vi "Red's Auto Clicker.vi"(8 "error in (no error)":errorcluster) -> (0 "error out":errorcluster)   [LabVIEW 2020]
doc: "Presents an interface to create, edit, save, and execute user-defined macros."
uses:
  CTLs/State Data.ctl
  CTLs/Macro Cluster V3.ctl
  CTLs/Macro Config V3.ctl
  CTLs/Step V3.ctl
  CTLs/Step Type V3.ctl
  CTLs/Hotkey Values.ctl
  CTLs/Refs.ctl
  <vilib>/Utility/miscctls.llb/LVRowAndColumnUnsignedTypeDef.ctl
  CTLs/FGV Actions.ctl
  CTLs/Hotkey Type.ctl
  fa5aba67-e91f-4216-ac5c-c17457851557.vi
  bd503c13-d10c-440e-ab5e-4e60baef5deb.vi
  <vilib>/Utility/inputDevices.llb/closeKeyboard.vi
  SubVIs/FaKI State Machine/FaKI State Machine.lvlib
panel:
  out "Status":string
  in  "Add Step 2":bool
  in  "Dbl Click":T1
  in  "Macro Steps":i32(listbox)
  out "Abort Hotkey":string caption="Abort Hotkey:"
  out "Metadata":string
  in  "Description":string
  out "Resolutions":cluster{"Width":i16, "Height":i16}[](array[cluster])
  out "n Monitors":i32
  in  "Settings":bool
  in  "Export":bool
  in  "Import":bool
  out "Macro Hotkey":string caption="Macro Hotkey:"
  in  "Delete":bool
  in  "Start/Stop":bool
  in  "N":i32 caption="Times to Repeat\n(-1 = indefinitely)" min=-1
  in  "Activation Type":enum32{"Hotkey", "Automatic"}(radio)
  out "Row":i32
  in  "Clear Steps":bool
  in  "Delete Step":bool
  in  "Insert Step":bool
  in  "Add Step":bool
  in  "Modify Step":bool
  in  "Exit":bool
  in  "Save":bool
  in  "Restore":bool
  in  "Help":bool
  in  "Macro Name":string(combo)
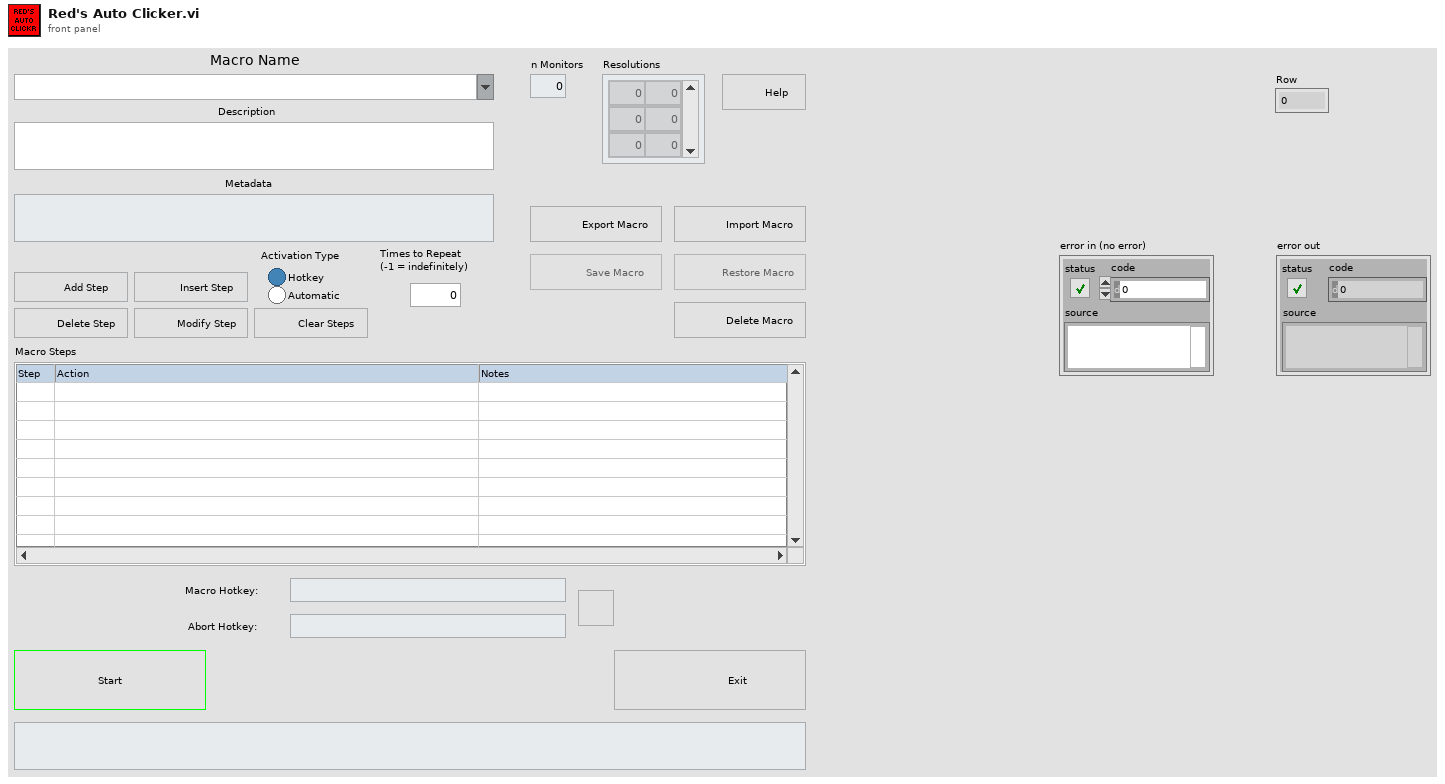
[diagram p1: front panel]
types:
  T1 = cluster{"Insert Before":bool, "Insert After":bool, "Modify Step 2":bool, "Delete Step 2":bool}
  T2 = typedef "LVPoint32TypeDef.ctl" = cluster{"Horizontal":i32, "Vertical":i32}
  T3 = enum32{"Invalid", "Standard", "Closed", "Hidden", "Minimized", "Maximized"}
  T4 = enum32{"invalid app kind", "Development System", "Run Time System", "Student Edition", "Embedded LabVIEW", "Evaluation", "Custom"}
  T5 = typedef "State Data.ctl" = cluster{"Core":cluster{"Current VI Reference":refnum<vi>, "Close Panel on Exit?":bool}, "Macro":cluster{"New":T6, "Saved":T6, "Name":string}, "Step":i32, "n":i32, "Hotkey Values":T10, "Keyboard":refnum<k1>, "Macro Active?":bool, "Macro Names":string[], "Rcount":i32, "Refs":T11, "Resolutions":cluster{"Width":i16, "Height":i16}[], "App Data Dir":path, "Start Time":timestamp}
  T6 = typedef "Macro Cluster V3.ctl" = cluster{"Config":T7, "Steps":T8[]}
  T7 = typedef "Macro Config V3.ctl" = cluster{"Schema Version":string, "Activation Type":enum32{"Hotkey", "Automatic"}, "N":i32, "Description":string, "Resolutions":cluster{"Width":i16, "Height":i16}[], "Date Created":timestamp, "Date Updated":timestamp}
  T8 = typedef "Step V3.ctl" = cluster{"Type":T9, "X":i32, "Y":i32, "Delay":i32, "Key":u8, "Repeat":i32, "RClick?":bool, "App/Window Name":string, "Notes":string}
  T9 = typedef "Step Type V3.ctl" = enum16{"Mouse Move", "Mouse Click", "Key Press", "Wait", "Mouse Down", "Mouse Up", "Key Down", "Key Up", "Run Application", "Maximize Window", "Restore Window", "Minimize Window", "Close Window", "Bring Window to Front", "Send Window to Back"}
  T10 = typedef "Hotkey Values.ctl" = cluster{"Macro Hotkey":enum16{"0", "1", "2", "3", "4", "5", "6", "7", "8", "9", "A", "B", "C", "D", "E", "F", "G", "H", "I", "J", "K", "L", "M", "N", "O", "P", "Q", "R", "S", "T", "U", "V", "W", "X", "Y", "Z", "F1", "F2", "F3", "F4", "F5", "F6", "F7", "F8", "F9", "F10", "F11", "F12", "F13", "F14", "F15", "ADD", "BACK", "BACKSLASH", "CAPITAL", "COMMA", "DECIMAL", "DELETE", "DIVIDE", "DOWN", "END", "EQUALS", "ESCAPE", "GRAVE (`)", "HOME", "INSERT", "LBRACKET", "LCONTROL", "LEFT", "L ALT", "LSHIFT", "LWIN", "MINUS", "MULTIPLY", "NEXT", "NUMLOCK", "NUMPAD_0", "NUMPAD_1", "NUMPAD_2", "NUMPAD_3", "NUMPAD_4", "NUMPAD_5", "NUMPAD_6", "NUMPAD_7", "NUMPAD_8", "NUMPAD_9", "PAUSE", "PERIOD", "PRIOR (PG UP)", "RBRACKET", "RCONTROL", "RETURN", "RIGHT", "R ALT", "RSHIFT", "RWIN", "SCROLL", "SEMICOLON", "SLASH", "SPACE", "SUBTRACT", "TAB", "UP", "ENTER (num pad)", "' (quote)"}[], "Abort Hotkey":enum16{"0", "1", "2", "3", "4", "5", "6", "7", "8", "9", "A", "B", "C", "D", "E", "F", "G", "H", "I", "J", "K", "L", "M", "N", "O", "P", "Q", "R", "S", "T", "U", "V", "W", "X", "Y", "Z", "F1", "F2", "F3", "F4", "F5", "F6", "F7", "F8", "F9", "F10", "F11", "F12", "F13", "F14", "F15", "ADD", "BACK", "BACKSLASH", "CAPITAL", "COMMA", "DECIMAL", "DELETE", "DIVIDE", "DOWN", "END", "EQUALS", "ESCAPE", "GRAVE (`)", "HOME", "INSERT", "LBRACKET", "LCONTROL", "LEFT", "L ALT", "LSHIFT", "LWIN", "MINUS", "MULTIPLY", "NEXT", "NUMLOCK", "NUMPAD_0", "NUMPAD_1", "NUMPAD_2", "NUMPAD_3", "NUMPAD_4", "NUMPAD_5", "NUMPAD_6", "NUMPAD_7", "NUMPAD_8", "NUMPAD_9", "PAUSE", "PERIOD", "PRIOR (PG UP)", "RBRACKET", "RCONTROL", "RETURN", "RIGHT", "R ALT", "RSHIFT", "RWIN", "SCROLL", "SEMICOLON", "SLASH", "SPACE", "SUBTRACT", "TAB", "UP", "ENTER (num pad)", "' (quote)"}[]}
  T11 = typedef "Refs.ctl" = cluster{"Name":refnum<vi>, "Description":refnum<vi>, "Import":refnum<vi>, "Export":refnum<vi>, "Delete":refnum<vi>, "Restore":refnum<vi>, "Save":refnum<vi>, "Start":refnum<vi>, "Steps":refnum<vi>, "Simple Refs":refnum<vi>[]}
  T12 = enum8{"Enabled", "Disabled", "Disabled and Grayed Out"}
  T13 = typedef "LVRowAndColumnUnsignedTypeDef.ctl" = cluster{"Row":u32, "Column":u32}
  T14 = typedef "Hotkey Type.ctl" = enum16{"Macro Hotkey", "Abort Hotkey"}
  T15 = typedef "FGV Actions.ctl" = enum16{"Read", "Write"}
  T16 = cluster{"Current VI Reference":refnum<vi>, "Close Panel on Exit?":bool}
  T17 = enum16{"0", "1", "2", "3", "4", "5", "6", "7", "8", "9", "A", "B", "C", "D", "E", "F", "G", "H", "I", "J", "K", "L", "M", "N", "O", "P", "Q", "R", "S", "T", "U", "V", "W", "X", "Y", "Z", "F1", "F2", "F3", "F4", "F5", "F6", "F7", "F8", "F9", "F10", "F11", "F12", "F13", "F14", "F15", "ADD", "BACK", "BACKSLASH", "CAPITAL", "COMMA", "DECIMAL", "DELETE", "DIVIDE", "DOWN", "END", "EQUALS", "ESCAPE", "GRAVE (`)", "HOME", "INSERT", "LBRACKET", "LCONTROL", "LEFT", "L ALT", "LSHIFT", "LWIN", "MINUS", "MULTIPLY", "NEXT", "NUMLOCK", "NUMPAD_0", "NUMPAD_1", "NUMPAD_2", "NUMPAD_3", "NUMPAD_4", "NUMPAD_5", "NUMPAD_6", "NUMPAD_7", "NUMPAD_8", "NUMPAD_9", "PAUSE", "PERIOD", "PRIOR (PG UP)", "RBRACKET", "RCONTROL", "RETURN", "RIGHT", "R ALT", "RSHIFT", "RWIN", "SCROLL", "SEMICOLON", "SLASH", "SPACE", "SUBTRACT", "TAB", "UP", "ENTER (num pad)", "' (quote)"}[]
  T18 = typedef "LVAllMonitorsDisplayTypeDef.ctl" = cluster{"Bounds":cluster{"Left":i16, "Top":i16, "Right":i16, "Bottom":i16}, "Depth":i16}[]
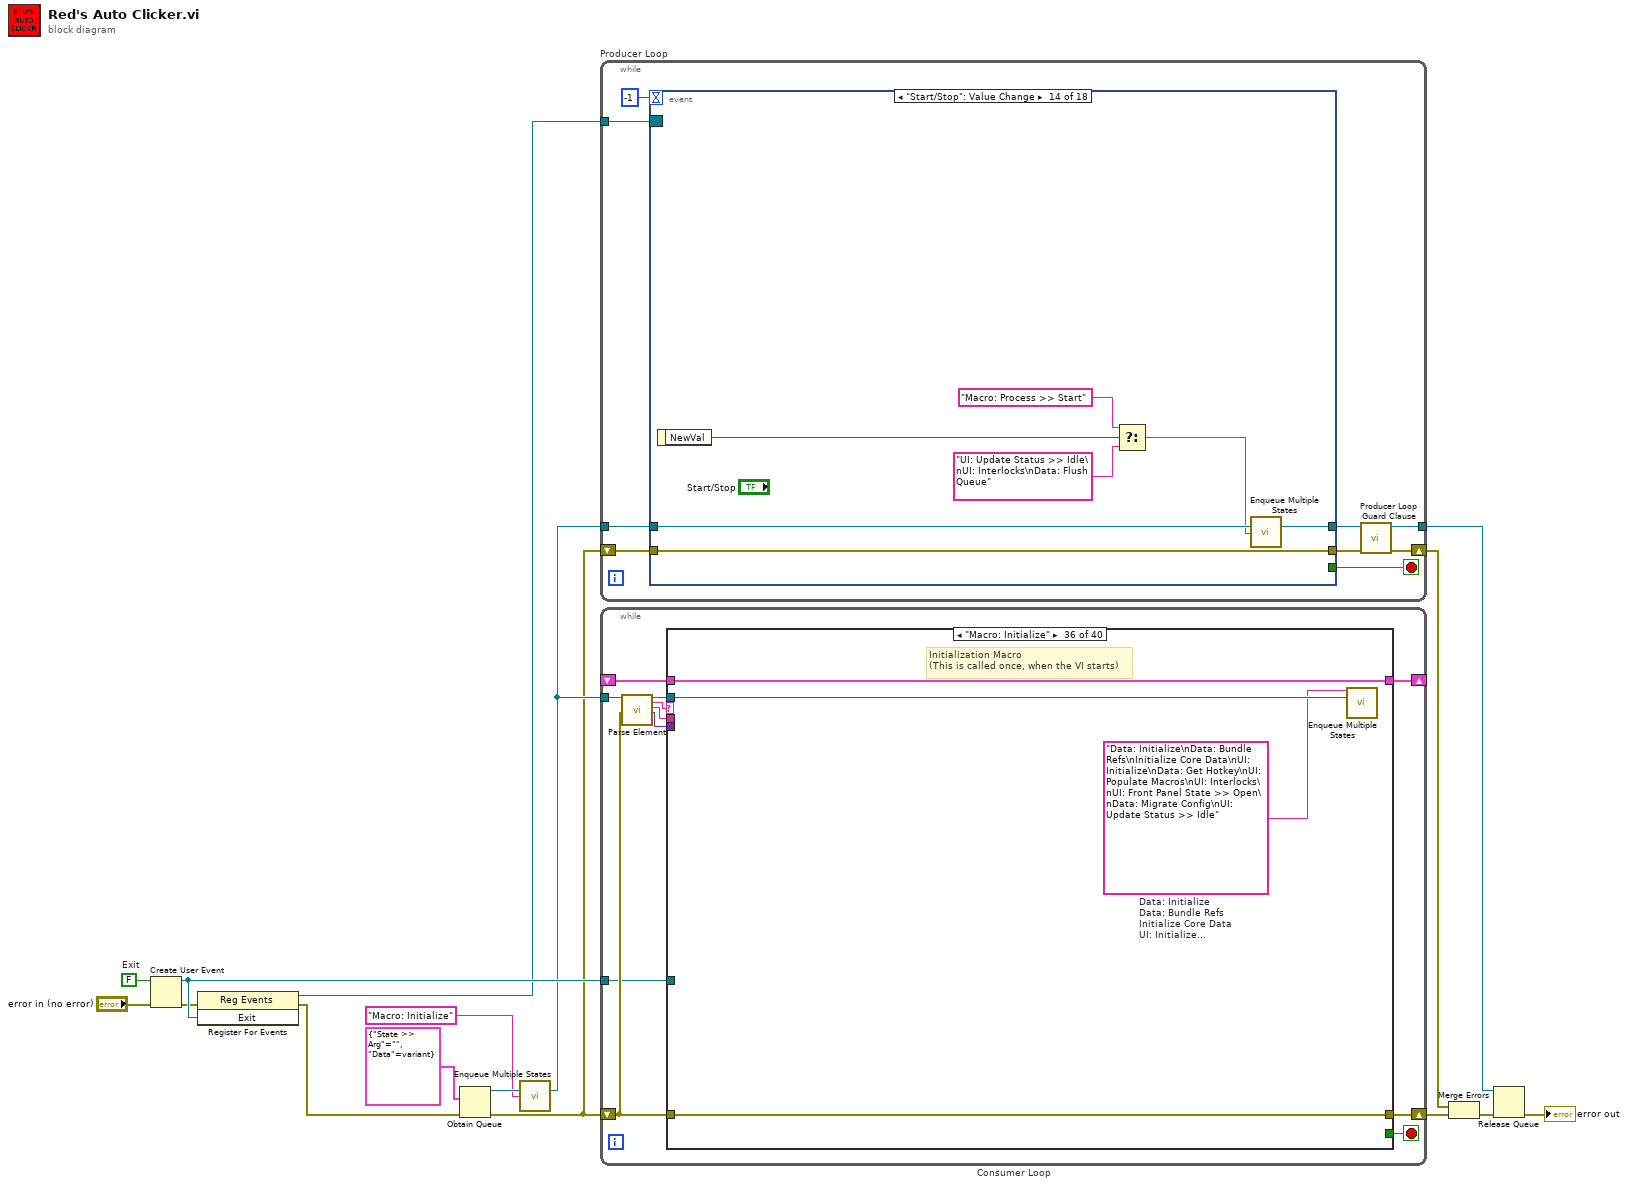
[diagram p0: block diagram]
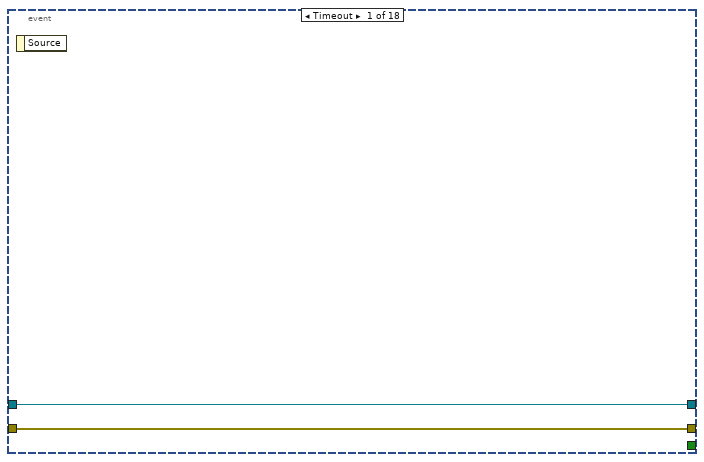
[diagram p2: hidden frame]
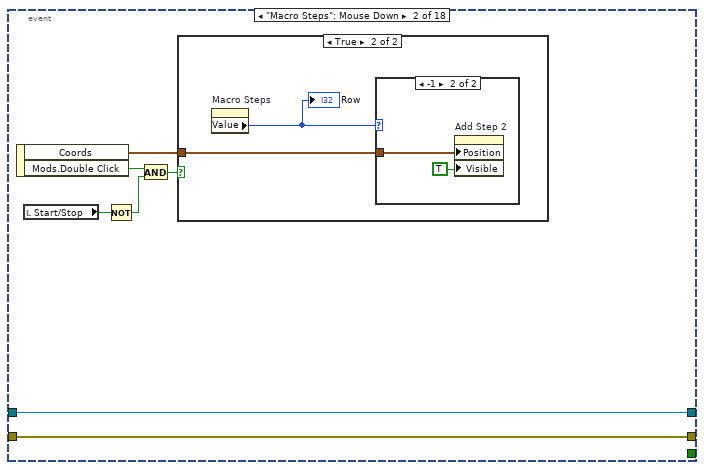
[diagram p3: hidden frame]
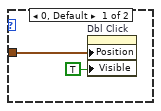
[diagram p5: hidden frame]
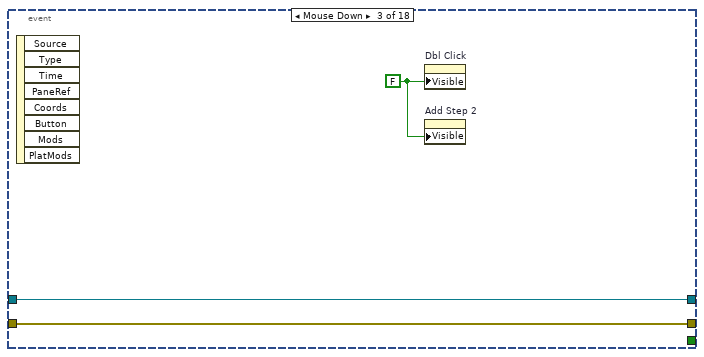
[diagram p6: hidden frame]
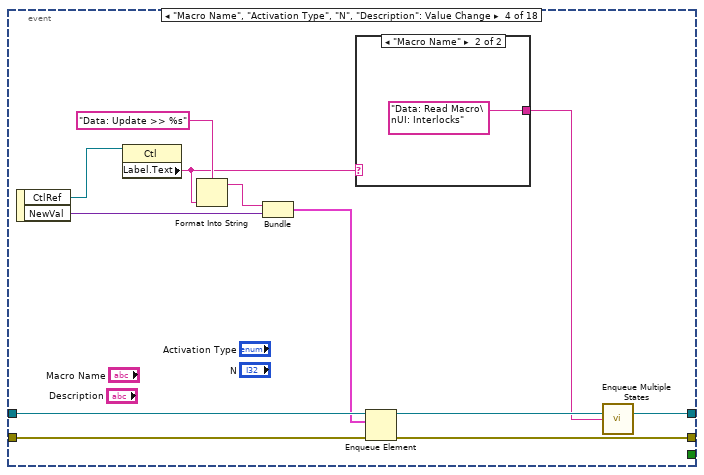
[diagram p7: hidden frame]
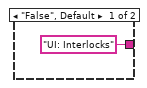
[diagram p8: hidden frame]
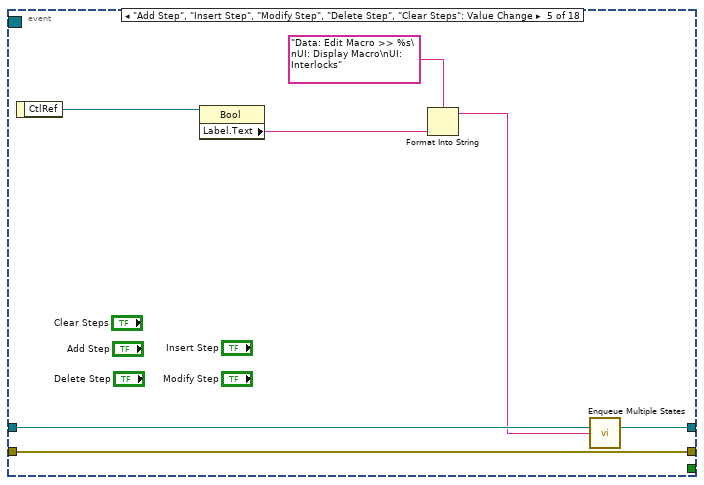
[diagram p9: hidden frame]
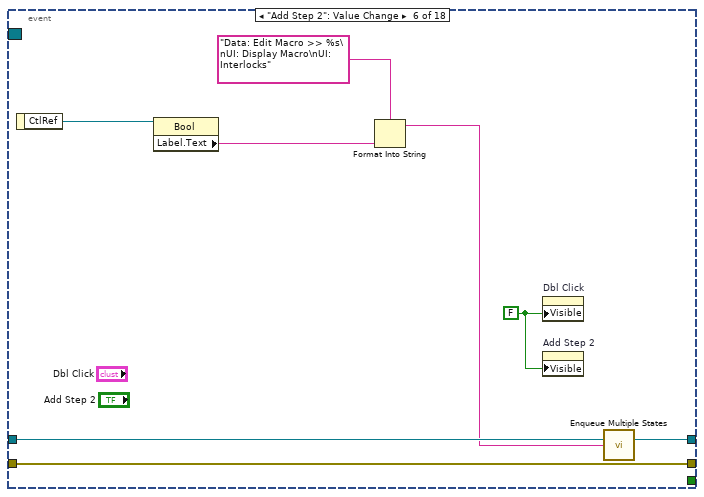
[diagram p10: hidden frame]
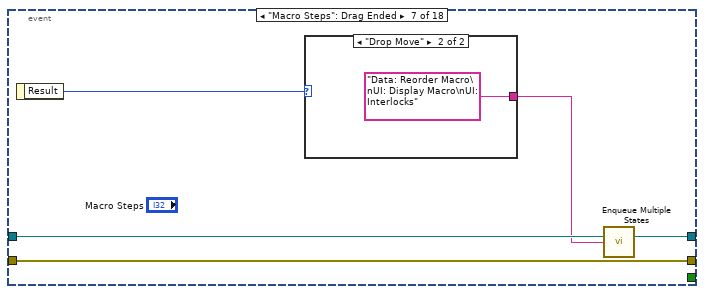
[diagram p11: hidden frame]
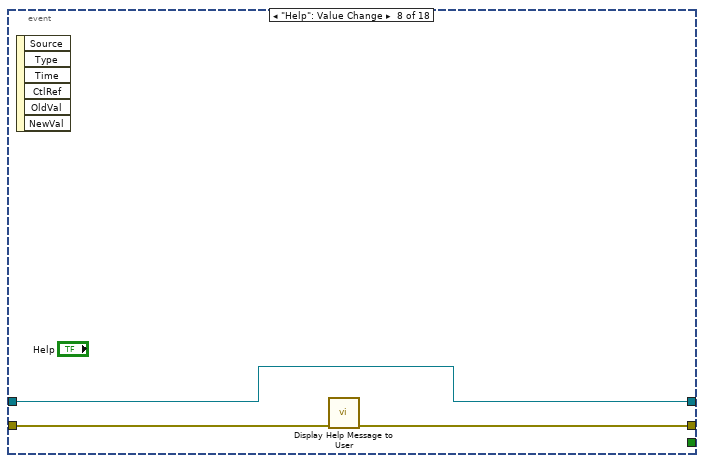
[diagram p13: hidden frame]
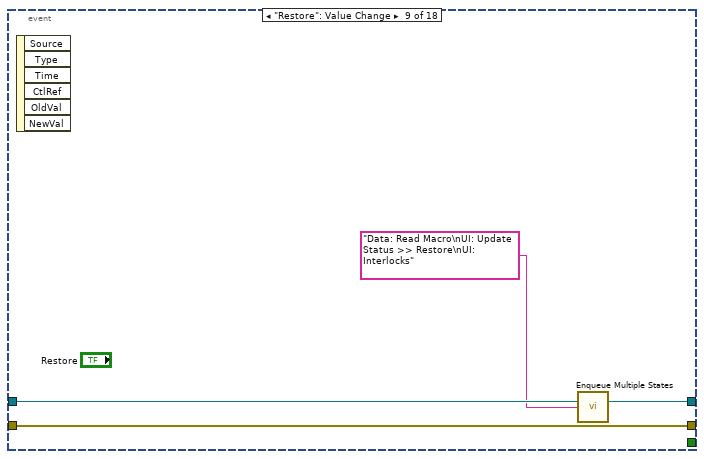
[diagram p14: hidden frame]
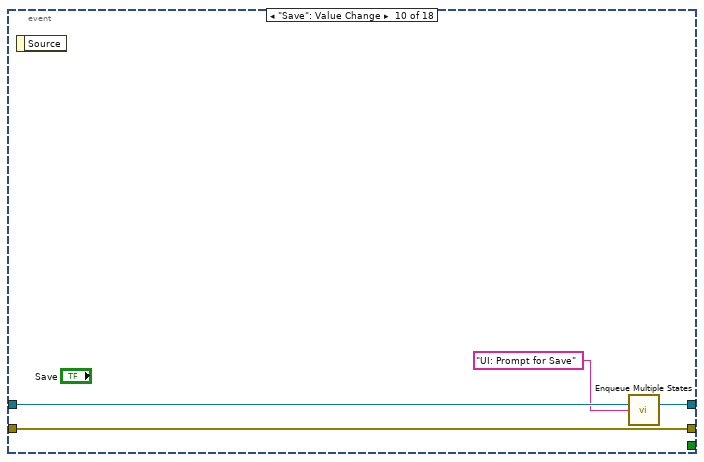
[diagram p15: hidden frame]
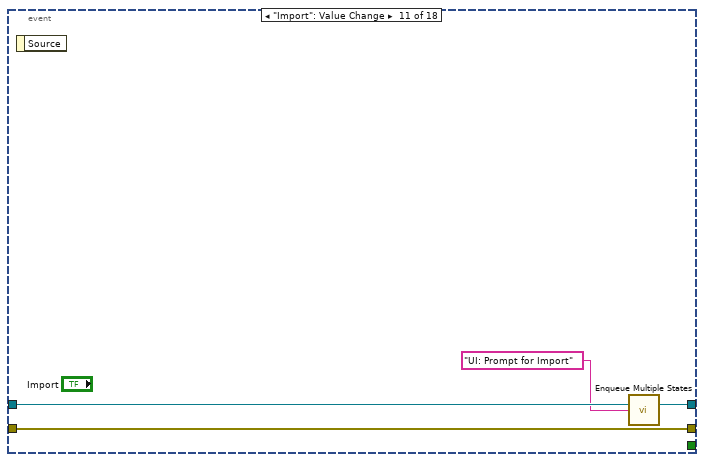
[diagram p16: hidden frame]
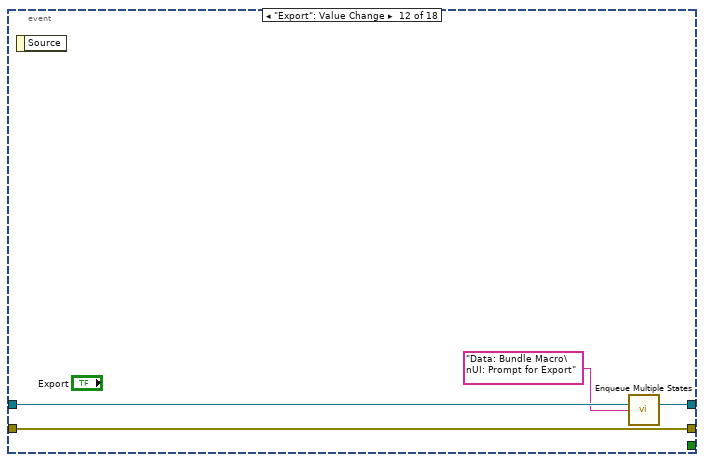
[diagram p17: hidden frame]
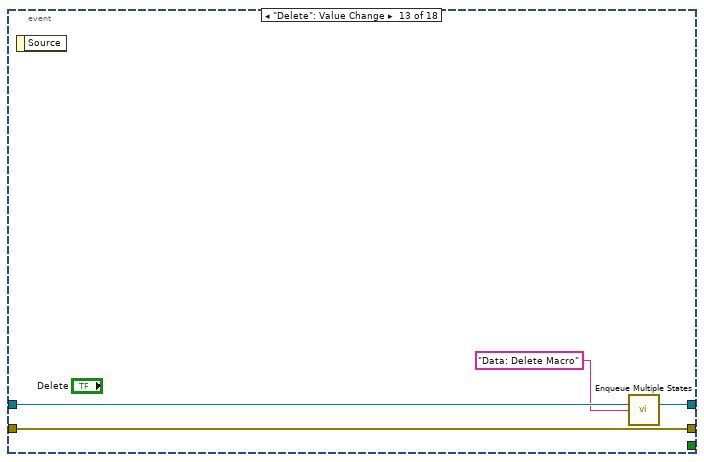
[diagram p18: hidden frame]
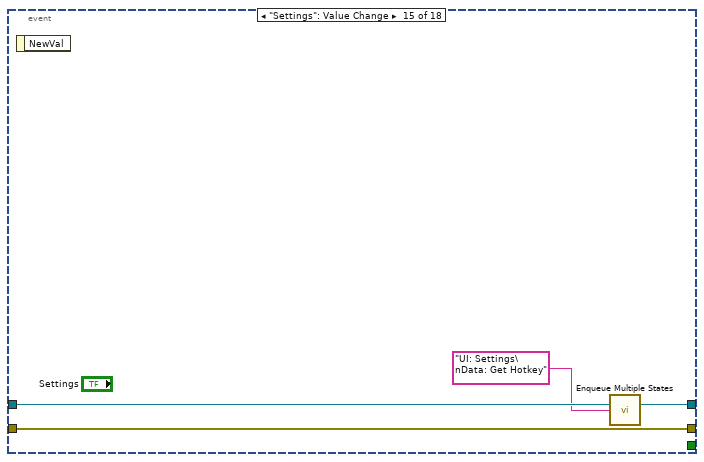
[diagram p19: hidden frame]
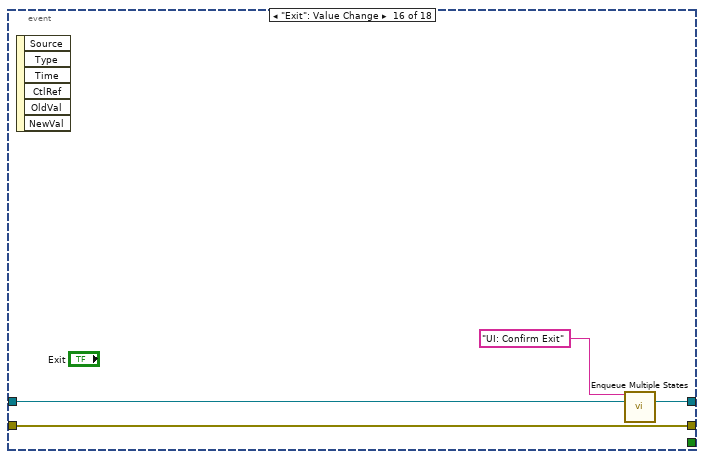
[diagram p20: hidden frame]
diagram:
  w13 = FALSE  # Exit
  n1 = Create User Event(user event datatype=w13, error in="error in (no error)") -> (user event=w16:refnum<user-event>, error out=w12:errorcluster)
  n2 = register-events(error in=w12, w16) -> (reference out=w15:refnum<event-registration>, error out=w14:errorcluster)  [unwired: 1 in]
  n3 = Obtain Queue(element data type=cluster{"State >> Arg":string, "Data":variant} {"State >> Arg"="", "Data"=variant}, error in (no error)=w14) -> (queue out=w6:refnum<queue>, error out=w3:errorcluster)  [unwired: 3 in, 1 out]
  n4 = call "Enqueue Multiple States.vi"("queue in"=w6, "State(s) at Back"="Macro: Initialize") -> ("queue out"=w7:refnum<queue>)  [unwired: 13 in]
  n5 = while "Producer Loop" {
    shift-right: [w25] -> w9
    shift-left: w3 -> [w23]
    tunnel: w15 -> [w19]
    tunnel: w7 -> [w21]
    tunnel: [w24] -> w11
    stop <- w18 stop-if-true
    n6 = event shown="[13] \"Start/Stop\": Value Change" {
      selector: w19 -> [_ _ _ _ _ _ _ _ _ _ _ _ _ _ _ _ _ _]
      dyn-events: _ -> [_ _ _ _ _ _ _ _ _ _ _ _ _ _ _ _ _ _]
      timeout: -1 ("Timeout") -> [_ _ _ _ _ _ _ _ _ _ _ _ _ _ _ _ _ _]
      tunnel: [w27 w34 w43 w51 w64 w72 w77 w80 w85 w89 w93 w97 w101 w108 w112 w116 w122 w127] -> w22
      tunnel: w23 -> [w27 w34 w43 w54 w64 w72 w77 w81 w85 w89 w93 w97 w101 w108 w112 w116 w122 w127]
      tunnel: w21 -> [w26 w32 w42 w48 w62 w69 w76 w79 w83 w88 w92 w96 w100 w104 w110 w114 w119 w125]
      tunnel: [w26 w32 w42 w53 w61 w68 w75 w79 w84 w87 w91 w95 w99 w105 w111 w113 w118 w124] -> w20
      tunnel: [_ _ _ _ _ _ _ _ _ _ _ _ _ _ _ _ FALSE TRUE] -> w18
      event Timeout {
        n7 = event-data() -> ()  [unwired: 1 in, 1 out]
      }
      event "Macro Steps": Mouse Down {
        n8 = event-data() -> ("Coords"=w33:T2, "Mods.Double Click"=w29:bool)  [unwired: 1 in]
        n9 = local read "Start/Stop"() -> (w31:bool)
        n10 = Not(x=w31) -> (.not. x?=w30:bool)
        n11 = And(x=w29, y=w30) -> (x .and. y?=w28:bool)
        n12 = case shown="True" w28 {
          tunnel: w33 -> [_ w36]
          frame False {
          }
          frame True {
            n13 = property on="Macro Steps" class="MCListbox (strict)"() -> ("Value"=w35:i32)  [unwired: 2 in, 2 out]
            "Row" <- w35
            n14 = case shown="-1" w35 {
              tunnel: w36 -> [w37 w39]
              frame 0, Default {
                n15 = property on="Dbl Click" class="Clust"("Position"=w37, "Visible"=TRUE) -> ()  [unwired: 2 in, 2 out]
              }
              frame -1 {
                n16 = property on="Add Step 2" class="Bool"("Position"=w39, "Visible"=TRUE) -> ()  [unwired: 2 in, 2 out]
              }
            }
          }
        }
      }
      event Mouse Down {
        w41 = FALSE ("Visible")
        n17 = event-data() -> ()  [unwired: 1 in, 8 out]
        n18 = property on="Dbl Click" class="Clust"("Visible"=w41) -> ()  [unwired: 2 in, 2 out]
        n19 = property on="Add Step 2" class="Bool"("Visible"=w41) -> ()  [unwired: 2 in, 2 out]
      }
      event "Macro Name", "Activation Type", "N", "Description": Value Change {
        n20 = event-data() -> ("CtlRef"=w50:refnum<vi>, "NewVal"=w46:variant)  [unwired: 1 in]
        n21 = property class="Ctl"(reference=w50) -> ("Label.Text"=w45:string)  [unwired: 1 in, 2 out]
        n22 = Format Into String(format string="Data: Update >> %s", w45) -> (resulting string=w47:string)  [unwired: 2 in, 1 out]
        n23 = Bundle(w47, "NewVal"=w46) -> (w44:cluster{string, "NewVal":variant})  [unwired: 1 in]
        n24 = case shown="\"Macro Name\"" w45 {
          tunnel: ["UI: Interlocks" ("string") "Data: Read Macro\nUI: Interlocks" ("string")] -> w52
          frame "False", Default {
          }
          frame "Macro Name" {
          }
        }
        n25 = Enqueue Element(queue=w48, element=w44, error in (no error)=w54) -> (queue out=w55:refnum<queue>, error out=w51:errorcluster)  [unwired: 1 in, 1 out]
        n26 = call "Enqueue Multiple States.vi"("queue in"=w55, "State(s) at Back"=w52) -> ("queue out"=w53:refnum<queue>)  [unwired: 13 in]
      }
      event "Add Step", "Insert Step", "Modify Step", "Delete Step", "Clear Steps": Value Change {
        n27 = event-data() -> ("CtlRef"=w63:refnum<vi>)  [unwired: 1 in]
        n28 = property class="Bool"(reference=w63) -> ("Label.Text"=w60:string)  [unwired: 1 in, 2 out]
        n29 = Format Into String(format string="Data: Edit Macro >> %s\nUI: Display Macro\nUI: Interlocks", w60) -> (resulting string=w58:string)  [unwired: 2 in, 1 out]
        n30 = call "Enqueue Multiple States.vi"("queue in"=w62, "State(s) at Back"=w58) -> ("queue out"=w61:refnum<queue>)  [unwired: 13 in]
      }
      event "Dbl Click.Insert Before", "Dbl Click.Insert After", "Dbl Click.Modify Step 2", "Dbl Click.Delete Step 2", "Add Step 2": Value Change {
        w70 = FALSE ("Visible")
        n31 = event-data() -> ("CtlRef"=w71:refnum<vi>)  [unwired: 1 in]
        n32 = property class="Bool"(reference=w71) -> ("Label.Text"=w66:string)  [unwired: 1 in, 2 out]
        n33 = Format Into String(format string="Data: Edit Macro >> %s\nUI: Display Macro\nUI: Interlocks", w66) -> (resulting string=w65:string)  [unwired: 2 in, 1 out]
        n34 = property on="Dbl Click" class="Clust"("Visible"=w70) -> ()  [unwired: 2 in, 2 out]
        n35 = property on="Add Step 2" class="Bool"("Visible"=w70) -> ()  [unwired: 2 in, 2 out]
        n36 = call "Enqueue Multiple States.vi"("queue in"=w69, "State(s) at Back"=w65) -> ("queue out"=w68:refnum<queue>)  [unwired: 13 in]
      }
      event "Macro Steps": Drag Ended {
        n37 = event-data() -> ("Result"=w73:enum16{"Drop Cancel", "Drop Move", "Drop Copy"})  [unwired: 1 in]
        n38 = case shown="\"Drop Move\"" w73 {
          tunnel: [_ "Data: Reorder Macro\nUI: Display Macro\nUI: Interlocks" ("State(s) at Back")] -> w74
          frame "Drop Cancel", Default {
          }
          frame "Drop Move" {
          }
        }
        n39 = call "Enqueue Multiple States.vi"("queue in"=w76, "State(s) at Back"=w74) -> ("queue out"=w75:refnum<queue>)  [unwired: 13 in]
      }
      event "Help": Value Change {
        n40 = event-data() -> ()  [unwired: 1 in, 6 out]
        n41 = call "Display Help Message to User"("error in (no error)"=w81) -> ("error out"=w80:errorcluster)  [unwired: 9 in, 1 out]
      }
      event "Restore": Value Change {
        n42 = event-data() -> ()  [unwired: 1 in, 6 out]
        n43 = call "Enqueue Multiple States.vi"("queue in"=w83, "State(s) at Back"="Data: Read Macro\nUI: Update Status >> Restore\nUI: Interlocks" ("State(s) at Back (\"\")")) -> ("queue out"=w84:refnum<queue>)  [unwired: 13 in]
      }
      event "Save": Value Change {
        n44 = event-data() -> ()  [unwired: 1 in, 1 out]
        n45 = call "Enqueue Multiple States.vi"("queue in"=w88, "State(s) at Back"="UI: Prompt for Save" ("State(s) at Back (\"\")")) -> ("queue out"=w87:refnum<queue>)  [unwired: 13 in]
      }
      event "Import": Value Change {
        n46 = event-data() -> ()  [unwired: 1 in, 1 out]
        n47 = call "Enqueue Multiple States.vi"("queue in"=w92, "State(s) at Back"="UI: Prompt for Import" ("State(s) at Back (\"\")")) -> ("queue out"=w91:refnum<queue>)  [unwired: 13 in]
      }
      event "Export": Value Change {
        n48 = event-data() -> ()  [unwired: 1 in, 1 out]
        n49 = call "Enqueue Multiple States.vi"("queue in"=w96, "State(s) at Back"="Data: Bundle Macro\nUI: Prompt for Export" ("State(s) at Back (\"\")")) -> ("queue out"=w95:refnum<queue>)  [unwired: 13 in]
      }
      event "Delete": Value Change {
        n50 = event-data() -> ()  [unwired: 1 in, 1 out]
        n51 = call "Enqueue Multiple States.vi"("queue in"=w100, "State(s) at Back"="Data: Delete Macro" ("State(s) at Back (\"\")")) -> ("queue out"=w99:refnum<queue>)  [unwired: 13 in]
      }
      event "Start/Stop": Value Change {
        n52 = event-data() -> ("NewVal"=w107:bool)  [unwired: 1 in]
        n53 = Select(t="Macro: Process >> Start", s=w107, f="UI: Update Status >> Idle\nUI: Interlocks\nData: Flush Queue") -> (s? t:f=w103:string)
        n54 = call "Enqueue Multiple States.vi"("queue in"=w104, "State(s) at Back"=w103) -> ("queue out"=w105:refnum<queue>)  [unwired: 13 in]
      }
      event "Settings": Value Change {
        n55 = event-data() -> ()  [unwired: 1 in, 1 out]
        n56 = call "Enqueue Multiple States.vi"("queue in"=w110, "State(s) at Back"="UI: Settings\nData: Get Hotkey" ("f")) -> ("queue out"=w111:refnum<queue>)  [unwired: 13 in]
      }
      event "Exit": Value Change {
        n57 = event-data() -> ()  [unwired: 1 in, 6 out]
        n58 = call "Enqueue Multiple States.vi"("State(s) at Front"="UI: Confirm Exit", "queue in"=w114) -> ("queue out"=w113:refnum<queue>)  [unwired: 13 in]
      }
      event Panel Close? {
        # "Discard the event because we'll close the front panel ourselves in Macro: Exit"
        n59 = event-data() -> ()  [unwired: 1 in, 1 out]
        n60 = call "Enqueue Multiple States.vi"("State(s) at Front"="UI: Confirm Exit", "queue in"=w119) -> ("queue out"=w118:refnum<queue>)  [unwired: 13 in]
        n61 = event-data("Discard?"=TRUE) -> ()  [unwired: 1 in, 1 out]
      }
      event User Event {
        n62 = event-data() -> ()  [unwired: 1 in, 5 out]
        n63 = call "Enqueue Multiple States.vi"("State(s) at Front"="Macro: Exit", "queue in"=w125) -> ("queue out"=w124:refnum<queue>)  [unwired: 13 in]
      }
    }
    n64 = call "Producer Loop Guard Clause.vi"("error in (no error)"=w22, "queue in"=w20) -> ("error out"=w25:errorcluster, "queue out"=w24:refnum<queue>)  [unwired: 8 in]
  }
  n65 = while "Consumer Loop" {
    shift-right: [w129] -> _
    shift-left: _ -> [w134]
    shift-right: [w136] -> w8
    shift-left: w3 -> [w137]
    tunnel: w7 -> [w138]
    tunnel: w16 -> [w128]
    stop <- w135 stop-if-true
    n66 = call "Parse Element.vi"("queue in"=w138, "error in (no error)"=w137) -> ("queue out"=w133:refnum<queue>, "State"=w132:string, "Arg"=w131:string, "Data"=w130:variant)  [unwired: 14 in]
    n67 = case shown="\"Macro: Initialize\"" w132 {
      selector: w132 -> [_ w141 _ _ _ _ _ _ _ _ _ _ _ _ _ _ _ _ _ _ _ _ _ _ _ _ _ _ _ _ _ _ _ _ _ _ _ _ _ _]
      tunnel: w133 -> [_ _ _ _ _ _ _ _ _ _ _ _ _ _ _ w351 w374 w387 _ _ _ _ _ _ _ _ _ w560 w575 _ w598 w610 w631 _ _ w657 w658 w730 _ w746]
      tunnel: w131 -> [_ _ _ w162 _ _ _ _ _ w215 _ w267 _ _ _ _ _ _ _ _ _ w415 w423 _ _ _ w513 _ _ _ _ _ _ _ _ _ w662 _ _ _]
      tunnel: w134 -> [w139 w143 w155 w165 w169 w170 _ w193 w205 w216 w265 w268 w318 w323 w339 w347 w371 w388 w396 w397 w401 w418 w425 w495 w500 w511 w514 w559 w578 w586 w597 w602 w623 w646 w652 w655 w659 w735 w737 w739]
      tunnel: [w140 w145 w159 errorcluster {"status"=FALSE, "code"=0, "source"=""} ("error out") w168 w171 w173 w194 w206 w211 w263 w270 w320 w330 w340 w349 w375 w389 w394 w398 w405 w416 w426 w496 w502 w506 w515 w553 w574 w584 w590 w603 w625 w640 w653 w656 w663 w736 w738 w744] -> w136
      tunnel: w137 -> [w140 w144 w159 w164 w168 w171 w179 w194 w204 w214 w257 w270 w320 w330 w341 w350 w376 w389 w393 w398 w405 w417 w427 w496 w503 w506 w515 w562 w579 w585 w590 w604 w626 w644 w653 w656 w663 w736 w738 w745]
      tunnel: [_ _ _ _ TRUE _ _ _ _ _ _ _ _ _ _ _ _ _ _ _ _ _ _ _ _ _ _ _ _ _ _ _ _ _ _ _ _ _ _ _] -> w135
      tunnel: w130 -> [_ _ _ w161 _ _ _ _ _ w213 _ _ _ _ _ _ _ _ _ _ _ _ _ _ _ _ _ _ _ _ _ _ _ _ _ _ _ _ _ _]
      tunnel: [w139 w143 w160 w165 w169 w170 w174 w192 w205 w212 w264 w269 w319 w329 w338 w348 w371 w388 w396 w397 w399 w418 w425 w495 w501 w511 w514 w559 w578 w586 w597 w601 w623 w646 w652 w655 w661 w735 w737 w739] -> w129
      tunnel: w128 -> [_ _ _ _ _ _ _ _ _ _ _ _ _ _ _ _ _ _ _ _ _ _ _ _ _ _ _ _ _ _ _ _ _ w638 _ _ _ _ _ _]
      frame "---------- Core ----------" {
        # "Do not put any code in this frame.\n(it is a separator no-op)"
      }
      frame Default {
        w148 = 42 items=["No error", "Argument error", "Memory is full", "Out of zone", "End of file", "File already open", "Generic file I/O error", "File not found", "File permission error", "Disk is full", "Duplicate path", "Too many files open", "System feature not enabled", "Resource file not found", "Cannot add resource", "Resource not found", "Image not found", "Image memory error", "Pen does not exist", "Config type invalid", "Config token not found", "Config parse error", "Config memory error", "Bad external code format", "Bad external code offset", "External code not present", "Null window", "Destroy window error", "Null menu", "Print aborted", "Bad print record", "Print driver error", "Windows error during printing", "Memory error during printing", "Print dialog error", "Generic print error", "Invalid device refnum", "Device not found", "Device parameter error", "Device unit error", "Cannot open device", "Device call aborted", "Generic error", "Cancelled by user", "Object ID too low", "Object ID too high", "Object not in heap", "Unknown heap", "Unknown object (invalid DefProc)", "Unknown object (DefProc not in table)", "Message out of range", "Invalid (null) method", "Unknown message", "Manager call not supported", "Bad address", "Network operation in progress", "Network operation timed out", "Connection is busy", "Network attribute not supported", "Network error", "Address in use", "System out of memory", "Connection aborted", "Connection refused", "Not connected", "Already connected", "Connection closed", "Initialization error (interapplication manager)", "Bad occurrence", "Wait on unbound occurrence handler", "Occurrence queue overflow", "Datalog type conflict", "Unused", "Unrecognized type (interapplication manager)", "Memory corrupt", "Failed to make temporary DLL", "Old CIN version", "Drag socket not found", "Failed to load drop-object", "Failed to register OLE object", "Failed to release OLE object", "Format specifier type mismatch", "Unknown format specifier", "Too few format specifiers", "Too many format specifiers", "Scan failed", "Newer CIN version", "Error converting to variant", "Runtime menu error", "Password tampered", "Variant attribute not found", "Incompatible variant data type", "Event data is not available", "Event Store is not present", "Occurrence is not found", "Event Queue is not created", "Event info is not available", "Refnum passed is NULL", "Error retrieving Class GUID", "Error retrieving CoClass GUID", "Error retrieving TypeLib GUID.", "Bad built application magic bytes.", "Specific driver is different from the specific driver associated with the Logical Name.", "There is no session opened to the class driver.", "Max Error", "MAX - Error with config objects", "MAX - Error loading configuration", "MAX - Group not supported"]
        # "Current State"
        # "Do not delete, rename, or modify this frame.\n(this is used to capture unhandled states and typos)"
        # "Handle mistyped state name (developer tool)"
        n68 = Format Into String(format string="Software Exception: Unhandled State \"%s\"." ("message"), error in=w144, w141) -> (resulting string=w147:string, error out=w146:errorcluster)  [unwired: 1 in]
        n69 = call <vilib>:"Error Cluster From Error Code.vi"("show call chain? (False)"=TRUE, "error in (no error)"=w146, "error message (\"\")"=w147, "error code (0)"=w148) -> ("error out"=w145:errorcluster)  [unwired: 5 in]
      }
      frame "Initialize Core Data" {
        # "Do not delete, rename, or modify this frame.\n(this is used to determine panel behavior on exit)"
        # "originally closed?"
        # "exe?"
        # "If panel starts closed or is an EXE, then close it when we exit"
        n70 = property class="VI"() -> ("FP.State"=w152:T3)  [unwired: 2 in, 2 out]
        n71 = property class="App"() -> ("App.Kind"=w158:T4)  [unwired: 2 in, 2 out]
        n72 = control-ref of="Current VI Reference"() -> (w153:refnum<vi>)
        n73 = Equal?(x=w152, y=T3."Closed" ("Front Panel Window:State")) -> (x = y?=w150:bool)
        n74 = Equal?(x=w158, y=T4."Run Time System" ("Application:Kind")) -> (x = y?=w156:bool)
        n75 = Or(x=w150, y=w156) -> (x .or. y?=w154:bool)
        n76 = Bundle By Name(cluster=w155, "Core.Current VI Reference"=w153, "Core.Close Panel on Exit?"=w154) -> (w160:T5)
      }
      frame "Error Handler" {
        # "Unhandled Error -- Display it"
        # "Handle any errors here.\nYou can also output any states to clean-up after errors occur"
        # "Clear error"
        n77 = call "Build Error Message.vi"("error in (no error)"=w164, "Data"=w161, "Arg"=w162) -> ("error out"=w163:errorcluster)  [unwired: 8 in]
        n78 = call <vilib>:"General Error Handler.vi"("error in (no error)"=w163) -> ()  [unwired: 10 in, 5 out]
      }
      frame "Exit" {
        # "Do not put any code in this frame.\n(No errors that occur here will be handled.)"
      }
      frame "---------- Data ----------" {
        # "Do not put any code in this frame.\n(It is a separator no-op. You can make a copy of this frame to create a new Data frame)"
      }
      frame "Data: Initialize" {
        w175 = T16 {"Current VI Reference"=refnum, "Close Panel on Exit?"=FALSE}  # Core
        # "Initialize the shift-register data, here."
        n79 = call <vilib>:"Intialize Keyboard.vi"("error in (no error)"=w179) -> ("error out"=w178:errorcluster, "device ID"=w176:refnum<k1>)  [unwired: 9 in]
        n80 = call "App Data Directory.vi"("error in (no error)"=w178) -> ("error out"=w173:errorcluster, "App Data Directory"=w172:path)  [unwired: 9 in]
        n81 = Bundle By Name(cluster=T5 {"Core"={"Current VI Reference"=refnum, "Close Panel on Exit?"=FALSE}, "Macro"={"New"={"Config"={"Schema Version"="", "Activation Type"=enum."Hotkey", "N"=0, "Description"="", "Resolutions"=[], "Date Created"=timestamp(0 s since 1904-01-01), "Date Updated"=timestamp(0 s since 1904-01-01)}, "Steps"=[]}, "Saved"={"Config"={"Schema Version"="", "Activation Type"=enum."Hotkey", "N"=0, "Description"="", "Resolutions"=[], "Date Created"=timestamp(0 s since 1904-01-01), "Date Updated"=timestamp(0 s since 1904-01-01)}, "Steps"=[]}, "Name"=""}, "Step"=0, "n"=0, "Hotkey Values"={"Macro Hotkey"=[], "Abort Hotkey"=[]}, "Keyboard"=refnum, "Macro Active?"=FALSE, "Macro Names"=[], "Rcount"=0, "Refs"={"Name"=refnum, "Description"=refnum, "Import"=refnum, "Export"=refnum, "Delete"=refnum, "Restore"=refnum, "Save"=refnum, "Start"=refnum, "Steps"=refnum, "Simple Refs"=[]}, "Resolutions"=[], "App Data Dir"=path "", "Start Time"=timestamp(0 s since 1904-01-01)}, "Core"=w175, "Keyboard"=w176, "App Data Dir"=w172) -> (w174:T5)
      }
      frame "Data: Bundle Refs" {
        n82 = control-ref of="Activation Type"() -> (w197:refnum<vi>)
        n83 = control-ref of="Macro Name"() -> (w195:refnum<vi>)
        n84 = control-ref of="Add Step"() -> (w202:refnum<vi>)
        n85 = control-ref of="Delete Step"() -> (w200:refnum<vi>)
        n86 = control-ref of="Insert Step"() -> (w199:refnum<vi>)
        n87 = control-ref of="Modify Step"() -> (w201:refnum<vi>)
        n88 = control-ref of="Clear Steps"() -> (w198:refnum<vi>)
        n89 = control-ref of="Settings"() -> (w183:refnum<vi>)
        n90 = control-ref of="Help"() -> (w181:refnum<vi>)
        n91 = control-ref of="N"() -> (w196:refnum<vi>)
        n92 = control-ref of="Macro Steps"() -> (w180:refnum<vi>)
        n93 = control-ref of="Macro Name"() -> (w191:refnum<vi>)
        n94 = control-ref of="Import"() -> (w189:refnum<vi>)
        n95 = control-ref of="Export"() -> (w188:refnum<vi>)
        n96 = control-ref of="Delete"() -> (w187:refnum<vi>)
        n97 = control-ref of="Restore"() -> (w186:refnum<vi>)
        n98 = control-ref of="Save"() -> (w185:refnum<vi>)
        n99 = control-ref of="Start/Stop"() -> (w184:refnum<vi>)
        n100 = control-ref of="Description"() -> (w190:refnum<vi>)
        n101 = Build Array(w202, w200, w199, w201, w198, w197, w196, w195, w183, w181) -> (w182:refnum<vi>[])
        n102 = Bundle By Name(cluster=w193, "Refs.Name"=w191, "Refs.Description"=w190, "Refs.Import"=w189, "Refs.Export"=w188, "Refs.Delete"=w187, "Refs.Restore"=w186, "Refs.Save"=w185, "Refs.Start"=w184, "Refs.Steps"=w180, "Refs.Simple Refs"=w182) -> (w192:T5)
      }
      frame "Data: Migrate Config" {
        n103 = Unbundle By Name(w205) -> ("App Data Dir"=w203:path)
        n104 = call "Config Paths.vi"("error in (no error)"=w204) -> ("error out"=w210:errorcluster, "Process Config"=w209:path, "Global Config"=w207:path)  [unwired: 8 in]
        n105 = call "Migrate Process Config.vi"("error in (no error)"=w210, "Old Process Config"=w209, "App Data Directory"=w203) -> ("error out"=w208:errorcluster)  [unwired: 8 in]
        n106 = call "Migrate Global Config.vi"("error in (no error)"=w208, "Old Global Config"=w207, "App Data Directory"=w203) -> ("error out"=w206:errorcluster)  [unwired: 8 in]
      }
      frame "Data: Update" {
        n107 = case shown="\"Macro Name\"" w215 {
          tunnel: w216 -> [w217 w222 w230 w237 w244 w251]
          tunnel: w214 -> [w218 w226 w233 w240 w247 w254]
          tunnel: w213 -> [_ w225 w232 w239 w246 w253]
          tunnel: [w217 w221 w229 w236 w243 w250] -> w212
          tunnel: [w218 w220 w228 w235 w242 w249] -> w211
          frame "False", Default {
          }
          frame "Macro Name" {
            n108 = Variant To Data(error in=w226, type="", Variant=w225) -> (data=w223:string, error out=w220:errorcluster)
            n109 = property on="Restore" class="Bool"("DisabledEnum"=T12."Disabled and Grayed Out" ("Disabled")) -> ()  [unwired: 2 in, 2 out]
            n110 = Bundle By Name(cluster=w222, "Macro.Name"=w223) -> (w221:T5)
          }
          frame "Activation Type" {
            n111 = Variant To Data(error in=w233, type=enum32{"Hotkey", "Automatic"}."Hotkey" ("FP CTLs.Type"), Variant=w232) -> (data=w231:enum32{"Hotkey", "Automatic"}, error out=w228:errorcluster)
            n112 = Bundle By Name(cluster=w230, "Macro.New.Config.Activation Type"=w231) -> (w229:T5)
          }
          frame "N" {
            n113 = Variant To Data(error in=w240, type=0 ("FP CTLs.N"), Variant=w239) -> (data=w238:i32, error out=w235:errorcluster)
            n114 = Bundle By Name(cluster=w237, "Macro.New.Config.N"=w238) -> (w236:T5)
          }
          frame "Description" {
            n115 = Variant To Data(error in=w247, type="" ("FP CTLs.N"), Variant=w246) -> (data=w245:string, error out=w242:errorcluster)
            n116 = Bundle By Name(cluster=w244, "Macro.New.Config.Description"=w245) -> (w243:T5)
          }
          frame "Macro Active?" {
            n117 = Variant To Data(error in=w254, type=FALSE, Variant=w253) -> (data=w252:bool, error out=w249:errorcluster)
            n118 = Bundle By Name(cluster=w251, "Macro Active?"=w252) -> (w250:T5)
          }
        }
      }
      frame "Data: Get Hotkey" {
        n119 = call "App Config INI.vi"("error in (no error)"=w257) -> ("error out"=w256:errorcluster, "App Config"=w255:path)  [unwired: 9 in]
        n120 = call "Get Hotkey.vi"("error in (no error)"=w256, "File Path"=w255) -> ("error out"=w263:errorcluster, "Hotkey Values"=w261:T10)  [unwired: 8 in]
        n121 = Unbundle By Name(w261) -> ("Macro Hotkey"=w260:T17, "Abort Hotkey"=w258:T17)
        n122 = Bundle By Name(cluster=w265, "Hotkey Values"=w261) -> (w264:T5)
        n123 = call "Convert Hotkey to String.vi"("Hotkey"=w260) -> ("String"=→"Macro Hotkey":string)  [unwired: 10 in]
        n124 = call "Convert Hotkey to String.vi"("Hotkey"=w258) -> ("String"=→"Abort Hotkey":string)  [unwired: 10 in]
      }
      frame "Data: Edit Macro" {
        n125 = local read "Row"() -> (w266:i32)
        n126 = in-place {
          in-place-border: w267 -> [w272]
          in-place-border: w266 -> [w271]
          n127 = in-place-cluster #1(w268) -> ("Macro.New.Steps"=w274:T8[])
          n128 = case shown="\"Add Step\"" w272 {
            tunnel: w274 -> [w275 w278 w281 w284 w287 w290 w294 w299 w303 w307 w309]
            tunnel: [w275 w277 w280 w283 w286 w289 w293 w298 w302 w306 w308] -> w273
            tunnel: w271 -> [_ _ _ _ _ _ w291 w296 w300 w304 _]
            frame Default {
            }
            frame "Add Step" {
              n129 = call "Alter Macro.vi"("Action"=enum16{"Add", "Insert", "Modify", "Delete"}."Add", "Steps in"=w278) -> ("Steps out"=w277:T8[])  [unwired: 9 in]
            }
            frame "Insert Step" {
              n130 = call "Alter Macro.vi"("Action"=enum16{"Add", "Insert", "Modify", "Delete"}."Insert", "Steps in"=w281) -> ("Steps out"=w280:T8[])  [unwired: 9 in]
            }
            frame "Modify Step" {
              n131 = call "Alter Macro.vi"("Action"=enum16{"Add", "Insert", "Modify", "Delete"}."Modify", "Steps in"=w284) -> ("Steps out"=w283:T8[])  [unwired: 9 in]
            }
            frame "Delete Step" {
              n132 = call "Alter Macro.vi"("Action"=enum16{"Add", "Insert", "Modify", "Delete"}."Delete", "Steps in"=w287) -> ("Steps out"=w286:T8[])  [unwired: 9 in]
            }
            frame "Add Step 2" {
              n133 = call "Alter Macro V2.vi"("Action"=enum16{"Add", "Insert", "Modify", "Delete"}."Add", "Steps in"=w290) -> ("Steps out"=w289:T8[])  [unwired: 9 in]
            }
            frame "Insert Before" {
              n134 = call "Alter Macro V2.vi"("Action"=enum16{"Add", "Insert", "Modify", "Delete"}."Insert", "Step"=w291, "Steps in"=w294) -> ("Steps out"=w293:T8[])  [unwired: 8 in]
            }
            frame "Insert After" {
              n135 = Increment(x=w296) -> (x+1=w295:i32)
              n136 = call "Alter Macro V2.vi"("Action"=enum16{"Add", "Insert", "Modify", "Delete"}."Insert", "Step"=w295, "Steps in"=w299) -> ("Steps out"=w298:T8[])  [unwired: 8 in]
            }
            frame "Modify Step 2" {
              n137 = call "Alter Macro V2.vi"("Action"=enum16{"Add", "Insert", "Modify", "Delete"}."Modify", "Step"=w300, "Steps in"=w303) -> ("Steps out"=w302:T8[])  [unwired: 8 in]
            }
            frame "Delete Step 2" {
              n138 = call "Alter Macro V2.vi"("Action"=enum16{"Add", "Insert", "Modify", "Delete"}."Delete", "Step"=w304, "Steps in"=w307) -> ("Steps out"=w306:T8[])  [unwired: 8 in]
            }
            frame "Clear Steps" {
              n139 = call "Confirm Clear"() -> ("OK"=w310:bool)  [unwired: 10 in, 1 out]
              n140 = case shown="False" w310 {
                tunnel: w309 -> [w311 _]
                tunnel: [w311 _] -> w308
                frame False {
                }
                frame True {
                  n141 = property on="Macro Steps" class="MCListbox (strict)"("TopLeft"=T13 {"Row"=0, "Column"=0} ("Index Values")) -> ()  [unwired: 2 in, 2 out]
                }
              }
            }
          }
          n142 = in-place-cluster #1("Macro.New.Steps"=w273) -> (w269:T5)
        }
      }
      frame "Data: Bundle Macro" {
        n143 = Unbundle By Name(w318) -> ("Resolutions"=w317:cluster{"Width":i16, "Height":i16}[], "Macro.New.Config.Date Created"=w315:timestamp)
        n144 = Get Date/Time In Seconds() -> (seconds since 1Jan1904=w313:timestamp)
        n145 = Not Equal To 0?(x=w315) -> (x != 0?=w316:bool)
        n146 = Select(t=w315, s=w316, f=w313) -> (s? t:f=w314:timestamp)
        n147 = Bundle By Name(cluster=w318, "Macro.New.Config.Resolutions"=w317, "Macro.New.Config.Date Created"=w314, "Macro.New.Config.Date Updated"=w313) -> (w319:T5)
      }
      frame "Data: Reorder Macro" {
        n148 = property on="Macro Steps" class="MCListbox (strict)"() -> ("ItemNames"=w328:string[][])  [unwired: 2 in, 2 out]
        n149 = Index Array(array=w328, index (col)=0 ("disabled index (col)")) -> (element=w326:string[])  [unwired: 1 in]
        n150 = Unbundle By Name(w323) -> ("Macro.New.Steps"=w322:T8[])
        n151 = Decimal String To Number(string=w326) -> (number=w325:i32[])  [unwired: 2 in, 1 out]
        n152 = Decrement(x=w325) -> (x-1=w324:i32[])
        n153 = for {
          tunnel: w324 -> [w331] mode=indexing
          tunnel: w322 -> [w333]
          tunnel: [w332] -> w321 mode=indexing
          n154 = Index Array(array=w333, index=w331) -> (element=w332:T8)
        }
        n155 = Bundle By Name(cluster=w323, "Macro.New.Steps"=w321) -> (w329:T5)
      }
      frame "Data: Save Macro" {
        n156 = Unbundle By Name(w339) -> ("Macro.New"=w337:T6, "App Data Dir"=w336:path, "Macro.Name"=w335:string)
        n157 = call "Build Path to Macro.vi"("Macro Name"=w335, "App Data Dir"=w336) -> ("Macro File Path"=w334:path)  [unwired: 9 in]
        n158 = call "Save Macro.vi"("error in (no error)"=w341, "Macro Cluster"=w337, "File Path"=w334) -> ("error out"=w340:errorcluster)  [unwired: 8 in]
        n159 = Bundle By Name(cluster=w339, "Macro.Saved"=w337) -> (w338:T5)
      }
      frame "Data: Read Macro" {
        n160 = Unbundle By Name(w347) -> ("Macro Names"=w346:string[], "Macro.Name"=w345:string, "App Data Dir"=w342:path)
        n161 = Search 1D Array(1D array=w346, element=w345) -> (index of element=w344:i32)  [unwired: 1 in]
        n162 = in-place {
          in-place-border: w350 -> [w360]
          in-place-border: [w359] -> w349
          in-place-border: w345 -> [w358]
          in-place-border: w344 -> [w357]
          in-place-border: w342 -> [w353]
          n163 = in-place-cluster #2(w347) -> ("Macro.New"=w356:T6)  [unwired: 1 out]
          n164 = case shown="0, Default" w357 {
            tunnel: w360 -> [w366 w369]
            tunnel: [w365 w369] -> w359
            tunnel: w358 -> [w362 _]
            tunnel: w356 -> [_ w368]
            tunnel: [w364 _] -> w355
            tunnel: [w364 w367] -> w354
            tunnel: w353 -> [w363 _]
            frame 0, Default {
              n165 = call "Build Path to Macro.vi"("Macro Name"=w362, "App Data Dir"=w363) -> ("Macro File Path"=w361:path)  [unwired: 9 in]
              n166 = call "Read Macro.vi"("error in (no error)"=w366, "File Path"=w361) -> ("error out"=w365:errorcluster, "Macro"=w364:T6)  [unwired: 8 in]
            }
            frame -1 {
              n167 = call "Clear Macro Data.vi"("Macro"=w368) -> ("Macro out"=w367:T6)  [unwired: 10 in]
            }
          }
          n168 = in-place-cluster #2("Macro.New"=w354, "Macro.Saved"=w355) -> (w348:T5)
        }
        n169 = property on="Macro Steps" class="MCListbox (strict)"("TopLeft"=T13 {"Row"=0, "Column"=0} ("Index Values")) -> ()  [unwired: 2 in, 2 out]
        n170 = call "Enqueue Multiple States.vi"("queue in"=w351, "State(s) at Back"="UI: Display Macro" ("State(s) at Back (\"\")")) -> ()  [unwired: 13 in, 1 out]
      }
      frame "Data: Delete Macro" {
        n171 = Unbundle By Name(w371) -> ("Macro.Name"=w372:string, "App Data Dir"=w370:path)
        n172 = call "Perm Delete?"("error in (no error)"=w376) -> ("error out"=w377:errorcluster, "Delete"=w378:bool)  [unwired: 9 in]
        n173 = case shown="True" w378 {
          tunnel: w377 -> [w379 w381]
          tunnel: [w379 w385] -> w375
          tunnel: [_ "UI: Update Status >> Delete\nUI: Populate Macros" ("State(s) at Back (\"\")")] -> w373
          tunnel: w372 -> [_ w383]
          tunnel: w370 -> [_ w382]
          frame False {
          }
          frame True {
            n174 = call "Delete Macro.vi"("Macro Name"=w383, "error in (no error)"=w381, "App Data Directory"=w382) -> ("error out"=w386:errorcluster)  [unwired: 8 in]
            n175 = property on="Macro Name" class="CmbBox"(error in=w386, "Val(Sgnl)"="") -> (error out=w385:errorcluster)  [unwired: 1 in, 1 out]
          }
        }
        n176 = call "Enqueue Multiple States.vi"("queue in"=w374, "State(s) at Back"=w373) -> ()  [unwired: 13 in, 1 out]
      }
      frame "Data: Flush Queue" {
        n177 = Flush Queue(queue=w387) -> ()  [unwired: 1 in, 3 out]
      }
      frame "Data: Cleanup" {
        # "Cleanup any data and references, here.\n(this is called automatically, by the Macro: Exit)"
        n178 = Unbundle By Name(w396) -> ("Core.Current VI Reference"=w395:refnum<vi>, "Keyboard"=w390:refnum<k1>)
        n179 = Close Reference(reference=w395, error in (no error)=w393) -> (error out=w391:errorcluster)
        n180 = call-poly <vilib>:"Close Input Device.vi"("error in (no error)"=w391, "device ID"=w390) -> ("error out"=w392:errorcluster)  [unwired: 8 in]
        n181 = invoke class="VI" method="Default Vals.Reinit All"(error in=w392) -> (error out=w394:errorcluster)  [unwired: 2 in, 2 out]
      }
      frame "---------- UI ----------" {
        # "Do not put any code in this frame.\n(It is a separator no-op. You can make a copy of this frame to create a new UI frame)"
      }
      frame "UI: Initialize" {
        w406 = T12."Disabled and Grayed Out" ("Disabled")
        # "Initialize the User Interface, here.\n(this is called automatically, by the Macro: Init)"
        n182 = property class="App"() -> ("Disp.AllMonitors"=w402:T18)  [unwired: 2 in, 2 out]
        n183 = for {
          tunnel: w402 -> [w414] mode=indexing
          tunnel: [w413] -> w400 mode=indexing
          n184 = Unbundle By Name(w414) -> ("Bounds.Right"=w412:i16, "Bounds.Left"=w410:i16, "Bounds.Bottom"=w411:i16, "Bounds.Top"=w409:i16)
          n185 = Subtract(x=w412, y=w410) -> (x-y=w407:i16)
          n186 = Subtract(x=w411, y=w409) -> (x-y=w408:i16)
          n187 = Bundle(w407, w408) -> (w413:cluster{i16, i16})  [unwired: 1 in]
        }
        "Resolutions" <- w400
        n188 = Array Size(array=w402) -> (size(s)=→"n Monitors":i32)
        n189 = property on="Start/Stop" class="Bool (strict)"("DisabledEnum"=w406) -> ()  [unwired: 2 in, 2 out]
        n190 = property on="Restore" class="Bool"("DisabledEnum"=w406) -> ()  [unwired: 2 in, 2 out]
        n191 = property on="Save" class="Bool"("DisabledEnum"=w406) -> ()  [unwired: 2 in, 2 out]
        n192 = property on="Start/Stop" class="Bool (strict)"("Colors [4]"=cluster{u32, u32}[] [{65280, 65280}, {16711680, 16711680}, {4424887, 6618880}, {4424887, 16711680}, {4424887, 12648384}, {4424887, 16761024}]) -> ()  [unwired: 2 in, 2 out]
        n193 = Bundle By Name(cluster=w401, "Resolutions"=w400) -> (w399:T5)
      }
      frame "UI: Cursor Set" {
        # "Argument"
        # "Set and Unset Cursor Busy.\n(Usage: \"UI: Cursor Set >> Busy|Idle\")"
        n194 = case shown="\"Idle\", Default" w415 {
          tunnel: w417 -> [w420 w422]
          tunnel: [w419 w421] -> w416
          frame "Idle", Default {
            n195 = call <vilib>:"Unset Busy.vi"("error in (no error)"=w420) -> ("error out"=w419:errorcluster)  [unwired: 10 in]
          }
          frame "Busy" {
            n196 = call <vilib>:"Set Busy.vi"("error in (no error)"=w422) -> ("error out"=w421:errorcluster)  [unwired: 9 in, 1 out]
          }
        }
      }
      frame "UI: Front Panel State" {
        # "Argument"
        # "Set Front Panel Open or Closed\n(Usage: \"UI: Front Panel State >> Open|Close\")"
        n197 = Unbundle By Name(w425) -> ("Core.Current VI Reference"=w424:refnum<vi>)
        n198 = case shown="\"Open\", \"Standard\", Default" w423 {
          tunnel: w427 -> [w433 w448 w459 w472 w485]
          tunnel: [w435 w449 w461 w474 w487] -> w426
          tunnel: w424 -> [w434 w446 w460 w473 w486]
          frame "Open", "Standard", Default {
            w428 = T3."Standard" ("State")
            n199 = property class="VI"(reference=w434, error in=w433) -> (reference out=w431:refnum<vi>, error out=w432:errorcluster, "FP.State"=w430:T3)
            n200 = Not Equal?(x=w430, y=w428) -> (x != y?=w429:bool)
            n201 = case shown="True" w429 {
              tunnel: [w439 w441] -> w435
              tunnel: w432 -> [w438 w441]
              tunnel: w431 -> [w437 _]
              tunnel: w428 -> [w436 _]
              frame True {
                n202 = invoke class="VI" method="FP.Open"(reference=w437, error in=w438, "Activate"=TRUE, "State"=w436) -> (error out=w439:errorcluster)  [unwired: 1 in, 4 out]
              }
              frame False {
              }
            }
          }
          frame "Close", "Closed" {
            n203 = property class="VI"(reference=w446, error in=w448) -> (reference out=w445:refnum<vi>, error out=w447:errorcluster, "FP.State"=w443:T3)
            n204 = Not Equal?(x=w443, y=T3."Closed" ("Front Panel Window:State")) -> (x != y?=w442:bool)
            n205 = case shown="True" w442 {
              tunnel: [w450 w453] -> w449
              tunnel: w447 -> [w450 w452]
              tunnel: w445 -> [_ w451]
              frame False {
              }
              frame True {
                n206 = invoke class="VI" method="FP.Close"(reference=w451, error in=w452) -> (error out=w453:errorcluster)  [unwired: 1 in, 2 out]
              }
            }
          }
          frame "Hidden", "Hide" {
            w454 = T3."Hidden" ("State")
            n207 = property class="VI"(reference=w460, error in=w459) -> (reference out=w457:refnum<vi>, error out=w458:errorcluster, "FP.State"=w456:T3)
            n208 = Not Equal?(x=w456, y=w454) -> (x != y?=w455:bool)
            n209 = case shown="True" w455 {
              tunnel: [w465 w466] -> w461
              tunnel: w458 -> [w464 w466]
              tunnel: w457 -> [w463 _]
              tunnel: w454 -> [w462 _]
              frame True {
                n210 = invoke class="VI" method="FP.Open"(reference=w463, error in=w464, "State"=w462) -> (error out=w465:errorcluster)  [unwired: 2 in, 4 out]
              }
              frame False {
              }
            }
          }
          frame "Minimize", "Minimized" {
            w467 = T3."Minimized" ("State")
            n211 = property class="VI"(reference=w473, error in=w472) -> (reference out=w470:refnum<vi>, error out=w471:errorcluster, "FP.State"=w469:T3)
            n212 = Not Equal?(x=w469, y=w467) -> (x != y?=w468:bool)
            n213 = case shown="True" w468 {
              tunnel: [w478 w479] -> w474
              tunnel: w471 -> [w477 w479]
              tunnel: w470 -> [w476 _]
              tunnel: w467 -> [w475 _]
              frame True {
                n214 = invoke class="VI" method="FP.Open"(reference=w476, error in=w477, "State"=w475) -> (error out=w478:errorcluster)  [unwired: 2 in, 4 out]
              }
              frame False {
              }
            }
          }
          frame "Maximize", "Maximized" {
            w480 = T3."Maximized" ("State")
            n215 = property class="VI"(reference=w486, error in=w485) -> (reference out=w483:refnum<vi>, error out=w484:errorcluster, "FP.State"=w482:T3)
            n216 = Not Equal?(x=w482, y=w480) -> (x != y?=w481:bool)
            n217 = case shown="True" w481 {
              tunnel: [w491 w492] -> w487
              tunnel: w484 -> [w490 w492]
              tunnel: w483 -> [w489 _]
              tunnel: w480 -> [w488 _]
              frame True {
                n218 = invoke class="VI" method="FP.Open"(reference=w489, error in=w490, "State"=w488) -> (error out=w491:errorcluster)  [unwired: 2 in, 4 out]
              }
              frame False {
              }
            }
          }
        }
      }
      frame "UI: Interlocks" {
        n219 = Unbundle By Name(w495) -> ("Refs"=w494:T11, "Macro"=w493:cluster{"New":T6, "Saved":T6, "Name":string})
        n220 = call "UI Interlocks.vi"("Macro"=w493, "Refs"=w494) -> ()  [unwired: 10 in]
      }
      frame "UI: Populate Macros" {
        n221 = Unbundle By Name(w500) -> ("App Data Dir"=w498:path)
        n222 = call "Read Macro Names.vi"("error in (no error)"=w503, "App Data Directory"=w498) -> ("error out"=w502:errorcluster, "Macro Names"=w499:string[])  [unwired: 8 in]
        n223 = Sort 1D Array(array=w499) -> (sorted array=w497:string[])
        n224 = Bundle By Name(cluster=w500, "Macro Names"=w497) -> (w501:T5)
        n225 = property on="Macro Name" class="CmbBox"("Strings[]"=w497) -> ()  [unwired: 2 in, 2 out]
      }
      frame "UI: Display Macro" {
        n226 = Unbundle By Name(w511) -> ("Macro.New"=w510:T6, "Macro.New.Config.Description"=w509:string, "Macro.New.Config.Activation Type"=w508:enum32{"Hotkey", "Automatic"}, "Macro.New.Config.N"=w507:i32)
        n227 = call "Display Data to Table.vi"("Macro"=w510) -> ("Metadata"=→"Metadata":string, "Macro Steps"=w504:string[][])  [unwired: 9 in]
        n228 = local write "Description"(w509) -> ()
        n229 = local write "Activation Type"(w508) -> ()
        n230 = local write "N"(w507) -> ()
        n231 = property on="Macro Steps" class="MCListbox (strict)"("ItemNames"=w504) -> ()  [unwired: 2 in, 2 out]
      }
      frame "UI: Update Status" {
        n232 = case shown="\"Abort Listen\"" w513 {
          tunnel: w514 -> [_ _ w524 w530 w536 w542 w548 _ _ _]
          tunnel: ["Idle" "Listening for hotkey press" w518 w525 w531 w537 w543 "Macro saved" ("Status") "Macro deleted" ("Status") "Macro restored to last save" ("Status")] -> w512
          frame "Idle", Default {
          }
          frame "Listen" {
          }
          frame "Step" {
            n233 = Unbundle By Name(w524) -> ("Macro.New"=w523:T6, "Step"=w522:i32, "n"=w521:i32, "Rcount"=w520:i32, "Start Time"=w519:timestamp)
            n234 = call "Build Status Message.vi"("Start Time"=w519, "Step Repeat"=w520, "Macro Repeat"=w521, "Step"=w522, "Macro"=w523) -> ("Status"=w518:string)  [unwired: 6 in]
          }
          frame "Complete Idle" {
            n235 = Unbundle By Name(w530) -> ("Start Time"=w528:timestamp)
            n236 = Get Date/Time In Seconds() -> (seconds since 1Jan1904=w527:timestamp)
            n237 = Subtract(x=w527, y=w528) -> (x-y=w526:dbl)
            n238 = Format Into String(format string="Macro completed in %.3t s.\nIdle", w526) -> (resulting string=w525:string)  [unwired: 2 in, 1 out]
          }
          frame "Complete Listen" {
            n239 = Unbundle By Name(w536) -> ("Start Time"=w534:timestamp)
            n240 = Get Date/Time In Seconds() -> (seconds since 1Jan1904=w533:timestamp)
            n241 = Subtract(x=w533, y=w534) -> (x-y=w532:dbl)
            n242 = Format Into String(format string="Macro completed in %.3t s.\nListening for hotkey press", w532) -> (resulting string=w531:string)  [unwired: 2 in, 1 out]
          }
          frame "Abort Idle" {
            n243 = Unbundle By Name(w542) -> ("Start Time"=w540:timestamp)
            n244 = Get Date/Time In Seconds() -> (seconds since 1Jan1904=w539:timestamp)
            n245 = Subtract(x=w539, y=w540) -> (x-y=w538:dbl)
            n246 = Format Into String(format string="Macro aborted after %.3t s.\nIdle", w538) -> (resulting string=w537:string)  [unwired: 2 in, 1 out]
          }
          frame "Abort Listen" {
            n247 = Unbundle By Name(w548) -> ("Start Time"=w546:timestamp)
            n248 = Get Date/Time In Seconds() -> (seconds since 1Jan1904=w545:timestamp)
            n249 = Subtract(x=w545, y=w546) -> (x-y=w544:dbl)
            n250 = Format Into String(format string="Macro aborted after %.3t s.\nListening for hotkey press", w544) -> (resulting string=w543:string)  [unwired: 2 in, 1 out]
          }
          frame "Save" {
          }
          frame "Delete" {
          }
          frame "Restore" {
          }
        }
        "Status" <- w512
      }
      frame "UI: Wait" {
        n251 = Unbundle By Name(w559) -> ("Keyboard"=w557:refnum<k1>, "Hotkey Values"=w556:T10)
        n252 = call "Check for Hotkey Press.vi"("Hotkey Type"=Hotkey_Type."Abort Hotkey", "error in (no error)"=w562, "Hotkeys"=w556, "Keyboard"=w557) -> ("error out"=w558:errorcluster, "Pressed?"=w554:bool)  [unwired: 5 in, 1 out]
        n253 = call "Timer FGV.vi"("Mode"=FGV_Actions."Read", "error in (no error)"=w558) -> ("error out"=w565:errorcluster, "Expired?"=w563:bool)  [unwired: 7 in, 1 out]
        n254 = case "Abort pressed?" shown="False" w554 {
          tunnel: w563 -> [w569 _]
          tunnel: [w566 "Macro: Process >> Abort" ("t")] -> w561
          frame False {
            n255 = Select(t="Macro: Process >> Count", s=w569, f="UI: Wait") -> (s? t:f=w566:string)
          }
          frame True {
          }
        }
        n256 = call "Stall Data Flow.vim"("value in"=w565, "milliseconds to wait"=u32 1) -> ("value out"=w553:errorcluster)  [unwired: 1 out]
        n257 = call "Enqueue Multiple States.vi"("queue in"=w560, "State(s) at Back"=w561) -> ()  [unwired: 13 in, 1 out]
      }
      frame "UI: Listen" {
        n258 = Unbundle By Name(w578) -> ("Keyboard"=w583:refnum<k1>, "Hotkey Values"=w573:T10)
        n259 = call "Stall Data Flow.vim"("value in"=w583, "milliseconds to wait"=u32 1) -> ("value out"=w581:refnum<k1>)  [unwired: 1 out]
        n260 = call "Check for Hotkey Press.vi"("Hotkey Type"=Hotkey_Type."Macro Hotkey", "error in (no error)"=w579, "Hotkeys"=w573, "Keyboard"=w581) -> ("error out"=w574:errorcluster, "Pressed?"=w571:bool)  [unwired: 5 in, 1 out]
        n261 = Select(t="Macro: Process >> Proc", s=w571, f="UI: Listen" ("string")) -> (s? t:f=w577:string)
        n262 = call "Enqueue Multiple States.vi"("queue in"=w575, "State(s) at Back"=w577) -> ()  [unwired: 13 in, 1 out]
      }
      frame "UI: Settings" {
        n263 = call "Change Settings.vi"("error in (no error)"=w585) -> ("error out"=w584:errorcluster)  [unwired: 10 in]
      }
      frame "UI: Prompt for Save" {
        n264 = Unbundle By Name(w597) -> ("Macro Names"=w589:string[], "Macro.Name"=w588:string)
        n265 = Search 1D Array(1D array=w589, element=w588) -> (index of element=w587:i32)  [unwired: 1 in]
        n266 = Greater Or Equal To 0?(x=w587) -> (x >= 0?=w593:bool)
        n267 = call "Overwrite?"("Enable"=w593) -> ("OK"=w592:bool)  [unwired: 9 in, 1 out]
        n268 = Implies(1:w592, 2:w593) -> (0:w591:bool)
        n269 = Select(t="Data: Bundle Macro\nData: Save Macro\nUI: Populate Macros\nUI: Update Status >> Save\nUI: Interlocks", s=w591, f="") -> (s? t:f=w594:string)
        n270 = call "Enqueue Multiple States.vi"("queue in"=w598, "State(s) at Back"=w594) -> ()  [unwired: 13 in, 1 out]
      }
      frame "UI: Prompt for Import" {
        n271 = call "File Dialog"("prompt"="Select a Macro to Import", "pattern (all files)"="*.ini", "pattern label"="Configuration Files") -> ("selected path"=w605:path, "cancelled"=w599:bool, "error out"=w611:errorcluster)  [unwired: 9 in, 1 out]
        n272 = case shown="False" w599 {
          tunnel: w605 -> [w615 _]
          tunnel: w604 -> [w614 w616]
          tunnel: [w613 w616] -> w603
          tunnel: [w612 _] -> w600
          frame False {
            n273 = call "Read Macro.vi"("error in (no error)"=w614, "File Path"=w615) -> ("error out"=w613:errorcluster, "Macro"=w612:T6)  [unwired: 8 in]
          }
          frame True {
          }
        }
        n274 = call <vilib>:"Clear Errors.vi"("error in (no error)"=w611) -> ()  [unwired: 5 in, 2 out]
        n275 = in-place {
          in-place-border: w600 -> [w619]
          in-place-border: w599 -> [w620]
          n276 = in-place-cluster #3(w602) -> ("Macro.New"=w618:T6)
          n277 = Select(t=w618, s=w620, f=w619) -> (s? t:f=w617:T6)
          n278 = in-place-cluster #3("Macro.New"=w617) -> (w601:T5)
        }
        n279 = call "Enqueue Multiple States.vi"("queue in"=w610, "State(s) at Back"="UI: Display Macro\nUI: Interlocks") -> ()  [unwired: 13 in, 1 out]
      }
      frame "UI: Prompt for Export" {
        n280 = Unbundle By Name(w623) -> ("Macro.New"=w621:T6, "Macro.Name"=w622:string)
        n281 = call "File Dialog2"("prompt"="Save As", "default name"=w622, "pattern (all files)"="*.ini", "pattern label"="Configuration Files") -> ("selected path"=w627:path, "cancelled"=w624:bool, "error out"=w632:errorcluster)  [unwired: 8 in, 1 out]
        n282 = case shown="False" w624 {
          tunnel: w627 -> [w636 _]
          tunnel: w626 -> [w635 w637]
          tunnel: [w634 w637] -> w625
          tunnel: w621 -> [w633 _]
          frame False {
            n283 = call "Save Macro.vi"("error in (no error)"=w635, "Macro Cluster"=w633, "File Path"=w636) -> ("error out"=w634:errorcluster)  [unwired: 8 in]
          }
          frame True {
          }
        }
        n284 = call <vilib>:"Clear Errors.vi"("error in (no error)"=w632) -> ()  [unwired: 5 in, 2 out]
        n285 = call "Enqueue Multiple States.vi"("queue in"=w631) -> ()  [unwired: 14 in, 1 out]
      }
      frame "UI: Confirm Exit" {
        n286 = Unbundle By Name(w646) -> ("Macro.New"=w642:T6, "Macro.Saved"=w643:T6)
        n287 = Not Equal?(x=w642, y=w643) -> (x != y?=w641:bool)
        n288 = call "Exit anyway?"("Enable"=w641) -> ("Exit"=w645:bool)  [unwired: 9 in, 1 out]
        n289 = Implies(1:w645, 2:w641) -> (0:w639:bool)
        n290 = case shown="True" w639 {
          tunnel: w644 -> [w647 w651]
          tunnel: [w647 w650] -> w640
          tunnel: w638 -> [_ w649]
          frame False {
          }
          frame True {
            n291 = Generate User Event(user event=w649, event data cluster=TRUE ("event data"), error in=w651) -> (error out=w650:errorcluster)  [unwired: 1 in, 1 out]
          }
        }
      }
      frame "---------- Macro ----------" {
        # "Do not put any code in this frame.\n(It is a separator no-op. You can make a copy of this frame to create a new Macro frame)"
      }
      frame "Macro: Initialize" {
        w654 = "Data: Initialize\nData: Bundle Refs\nInitialize Core Data\nUI: Initialize\nData: Get Hotkey\nUI: Populate Macros\nUI: Interlocks\nUI: Front Panel State >> Open\nData: Migrate Config\nUI: Update Status >> Idle"  # Data: Initialize Data: Bundle Refs Initialize Core Data UI: Initialize Data: Get Hotkey UI: Populate Macros UI: Interlocks UI: Front Panel State >> Open Data: Migrate Config UI: Update Status >> Idle
        # "Initialization Macro\n(This is called once, when the VI starts)"
        n292 = call "Enqueue Multiple States.vi"("State(s) at Front"=w654, "queue in"=w657) -> ()  [unwired: 13 in, 1 out]
      }
      frame "Macro: Process" {
        n293 = case shown="\"Count\"" w662 {
          tunnel: w659 -> [w665 w672 w681 w696 w708 w714 w716 w722]
          tunnel: [w665 w675 w679 w694 w706 w713 w716 w722] -> w661
          tunnel: [w664 "UI: Interlocks\nMacro: Process >> Step" w677 w692 w704 "UI: Update Status >> Step\nProcess: Perform Step" w717 w723] -> w660
          frame "Start", Default {
            # "Reached when Start button is pressed"
            n294 = Unbundle By Name(w665) -> ("Macro.New.Config.Activation Type"=w666:enum32{"Hotkey", "Automatic"})
            n295 = Equal?(x=w666, y=enum32{"Hotkey", "Automatic"}."Hotkey") -> (x = y?=w670:bool)
            n296 = Select(t="UI: Interlocks\nUI: Update Status >> Listen\nUI: Listen", s=w670, f="Macro: Proc") -> (s? t:f=w664:string)
          }
          frame "Proc" {
            w674 = 0 ("Step")
            # "Reached when Macro hotkey is activated or right after Start button for Automatic activation type"
            n297 = Get Date/Time In Seconds() -> (seconds since 1Jan1904=w673:timestamp)
            n298 = Bundle By Name(cluster=w672, "Step"=w674, "n"=w674, "Rcount"=w674, "Start Time"=w673) -> (w675:T5)
          }
          frame "Step" {
            # "Reached when a macro procs, or the current step of a macro finishes executing"
            n299 = Unbundle By Name(w681) -> ("Step"=w686:i32, "Macro.New.Steps"=w684:T8[])
            n300 = Array Size(array=w684) -> (size(s)=w685:i32)
            n301 = Increment(x=w686) -> (x+1=w680:i32)
            n302 = Greater Or Equal?(x=w680, y=w685) -> (x >= y?=w683:bool)
            n303 = Bundle By Name(cluster=w681, "Step"=w680, "Rcount"=0) -> (w679:T5)
            n304 = Select(t="Macro: Process >> End", s=w683, f="UI: Update Status >> Step\nProcess: Perform Step") -> (s? t:f=w677:string)
          }
          frame "Count" {
            # "Reached when one count of the current step of a macro finishes executing"
            n305 = Unbundle By Name(w696) -> ("Rcount"=w687:i32, "Macro.New.Steps"=w691:T8[], "Step"=w690:i32)
            n306 = Index Array(array=w691, index=w690) -> (element=w689:T8)
            n307 = Unbundle By Name(w689) -> ("Repeat"=w688:i32)
            n308 = Increment(x=w687) -> (x+1=w695:i32)
            n309 = Greater Or Equal?(x=w687, y=w688) -> (x >= y?=w698:bool)
            n310 = Bundle By Name(cluster=w696, "Rcount"=w695) -> (w694:T5)
            n311 = Select(t="Macro: Process >> Step", s=w698, f="UI: Update Status >> Step\nProcess: Perform Step") -> (s? t:f=w692:string)
          }
          frame "End" {
            # "Reached when the last step of a macro finishes executing"
            n312 = Unbundle By Name(w708) -> ("n"=w710:i32, "Macro.New.Config.N"=w699:i32)
            n313 = Increment(x=w710) -> (x+1=w707:i32)
            n314 = Greater?(x=w707, y=w699) -> (0:w702:bool)
            n315 = Not Equal?(x=w699, y=-1) -> (x != y?=w701:bool)
            n316 = And(x=w702, y=w701) -> (x .and. y?=w700:bool)
            n317 = Bundle By Name(cluster=w708, "n"=w707) -> (w706:T5)
            n318 = Select(t="Macro: Process >> Complete", s=w700, f="Macro: Process >> Repeat") -> (s? t:f=w704:string)
          }
          frame "Repeat" {
            w711 = 0 ("Step")
            # "Reached when a whole macro needs to be repeated"
            n319 = Bundle By Name(cluster=w714, "Step"=w711, "Rcount"=w711) -> (w713:T5)
          }
          frame "Complete" {
            # "Reached when a macro fully finishes including all repeats"
            n320 = Unbundle By Name(w716) -> ("Macro.New.Config.Activation Type"=w715:enum32{"Hotkey", "Automatic"})
            n321 = case shown="\"Hotkey\"" w715 {
              tunnel: ["UI: Update Status >> Complete Listen\nUI: Listen" "UI: Update Status >> Complete Idle"] -> w717
              frame "Hotkey" {
              }
              frame "Automatic" {
                n322 = property on="Start/Stop" class="Bool (strict)"("Val(Sgnl)"=FALSE ("Value (Signaling)")) -> ()  [unwired: 2 in, 2 out]
              }
            }
          }
          frame "Abort" {
            # "Reached when Abort hotkey is detected"
            n323 = Unbundle By Name(w722) -> ("Macro.New.Config.Activation Type"=w721:enum32{"Hotkey", "Automatic"})
            n324 = case shown="\"Automatic\"" w721 {
              tunnel: ["UI: Update Status >> Abort Listen\nUI: Listen" "UI: Update Status >> Abort Idle"] -> w723
              frame "Hotkey" {
              }
              frame "Automatic" {
                n325 = property on="Start/Stop" class="Bool (strict)"("Val(Sgnl)"=FALSE ("Value (Signaling)")) -> ()  [unwired: 2 in, 2 out]
              }
            }
          }
        }
        n326 = call "Enqueue Multiple States.vi"("queue in"=w658, "State(s) at Back"=w660) -> ()  [unwired: 13 in, 1 out]
      }
      frame "Macro: Exit" {
        # "Exit Macro\n(This is called once, when the VI exits)"
        n327 = Unbundle By Name(w735) -> ("Core.Close Panel on Exit?"=w734:bool)
        n328 = property on="Macro Steps" class="MCListbox (strict)"("TopLeft"=T13 {"Row"=0, "Column"=0} ("Index Values")) -> ()  [unwired: 2 in, 2 out]
        n329 = property on="Macro Steps" class="MCListbox (strict)"("ItemNames"=string[][] [] ("Item Names")) -> ()  [unwired: 2 in, 2 out]
        n330 = Select(t="UI: Front Panel State >> Close", s=w734, f="") -> (s? t:f=w729:string)
        n331 = call "Enqueue Multiple States.vi"("State(s) at Front"=w729, "queue in"=w730, "State(s) at Back"="Data: Cleanup\nExit") -> ()  [unwired: 12 in, 1 out]
      }
      frame "---------- Process ----------" {
      }
      frame "Process: Perform Step" {
        n332 = Unbundle By Name(w739) -> ("Macro.New.Steps"=w748:T8[], "Step"=w747:i32, "Hotkey Values"=w742:T10, "Keyboard"=w743:refnum<k1>)
        n333 = Index Array(array=w748, index=w747) -> (element=w741:T8)
        n334 = call "Perform Step.vi"("error in (no error)"=w745, "Keyboard"=w743, "Hotkeys"=w742, "Step"=w741) -> ("error out"=w744:errorcluster, "State(s)"=w740:string)  [unwired: 6 in]
        n335 = call "Enqueue Multiple States.vi"("queue in"=w746, "State(s) at Back"=w740) -> ()  [unwired: 13 in, 1 out]
      }
    }
  }
  n336 = Merge Errors(w9, w8) -> (w10:errorcluster)
  n337 = Release Queue(queue=w11, error in (no error)=w10) -> (error out=→"error out":errorcluster)  [unwired: 1 in, 2 out]
